vi "Settings Dialog.vi"(8 "error in (no error)":errorcluster, 11 "Settings In":T1={"Camera Configuration"={"Camera Index"=0}, "Logging Configuration"={"Log File Base Path"=path ""}, "XYZ Configuration"={"VISA resource name"="", "Timeout (3sec)"=0}, "DM Configuration"={"Selected Profile"="", "dm out"={"type"=0, "ID"=0, "size"=0, "@dummy control@"=0, "@dummy control@"=0, "@dummy control@"=0, "@dummy control@"=0, "lutName"=0}}, "Automation Configuration"={" Index"=0}, "V7001 Configuration"={" Index"=0}, "AOD Configuration"={"Physical Channel"="Dev1/ao0:1", "Maximum Value"=0.0, "Minimum Value"=1.0, "Update Rate"=192000.0}} {"AOD Configuration"."Update Rate" format="%0.2f"; "AOD Configuration"."Minimum Value" format="%0.2f"; "AOD Configuration"."Maximum Value" format="%0.2f"}) -> (0 "error out":errorcluster, 1 "Cancelled?":bool, 2 "UI Refresh Needed?":bool, 3 "Settings Out":T1={"Camera Configuration"={"Camera Index"=0}, "Logging Configuration"={"Log File Base Path"=path ""}, "XYZ Configuration"={"VISA resource name"="", "Timeout (3sec)"=0}, "DM Configuration"={"Selected Profile"="", "dm out"={"type"=0, "ID"=0, "size"=0, "@dummy control@"=0, "@dummy control@"=0, "@dummy control@"=0, "@dummy control@"=0, "lutName"=0}}, "Automation Configuration"={" Index"=0}, "V7001 Configuration"={" Index"=0}, "AOD Configuration"={"Physical Channel"="Dev1/ao0:1", "Maximum Value"=0.0, "Minimum Value"=1.0, "Update Rate"=192000.0}} {"AOD Configuration"."Update Rate" format="%0.2f"; "AOD Configuration"."Minimum Value" format="%0.2f"; "AOD Configuration"."Maximum Value" format="%0.2f"})   [LabVIEW 2015, in "Settings.lvlib"]
uses:
  Settings.lvlib
  <vilib>/Utility/xml.llb/Write to XML File(string).vi
  Camera/Camera Configuration.ctl
  Camera/Camera.lvlib
  Logging/Logging Configuration.ctl
  Logging/Logging.lvlib
  Settings.ctl
  XYZStage/XYZStage Configuration.ctl
  XYZStage/XYZStage.lvlib
  DM/DM Configuration.ctl
  DM/DM.lvlib
  Automation/Automation Configuration.ctl
  Automation/Automation.lvlib
  V7001/V7001 Configuration.ctl
  V7001/V7001.lvlib
  AOD/AOD Configuration.ctl
  AOD/AOD.lvlib
panel:
  in  "Cancel Button":bool
  in  "OK Button":bool
  in  "Log File Path":path
  in  "Signal Type":u16(ring) items=["Sine Wave", "Square with Noise"]
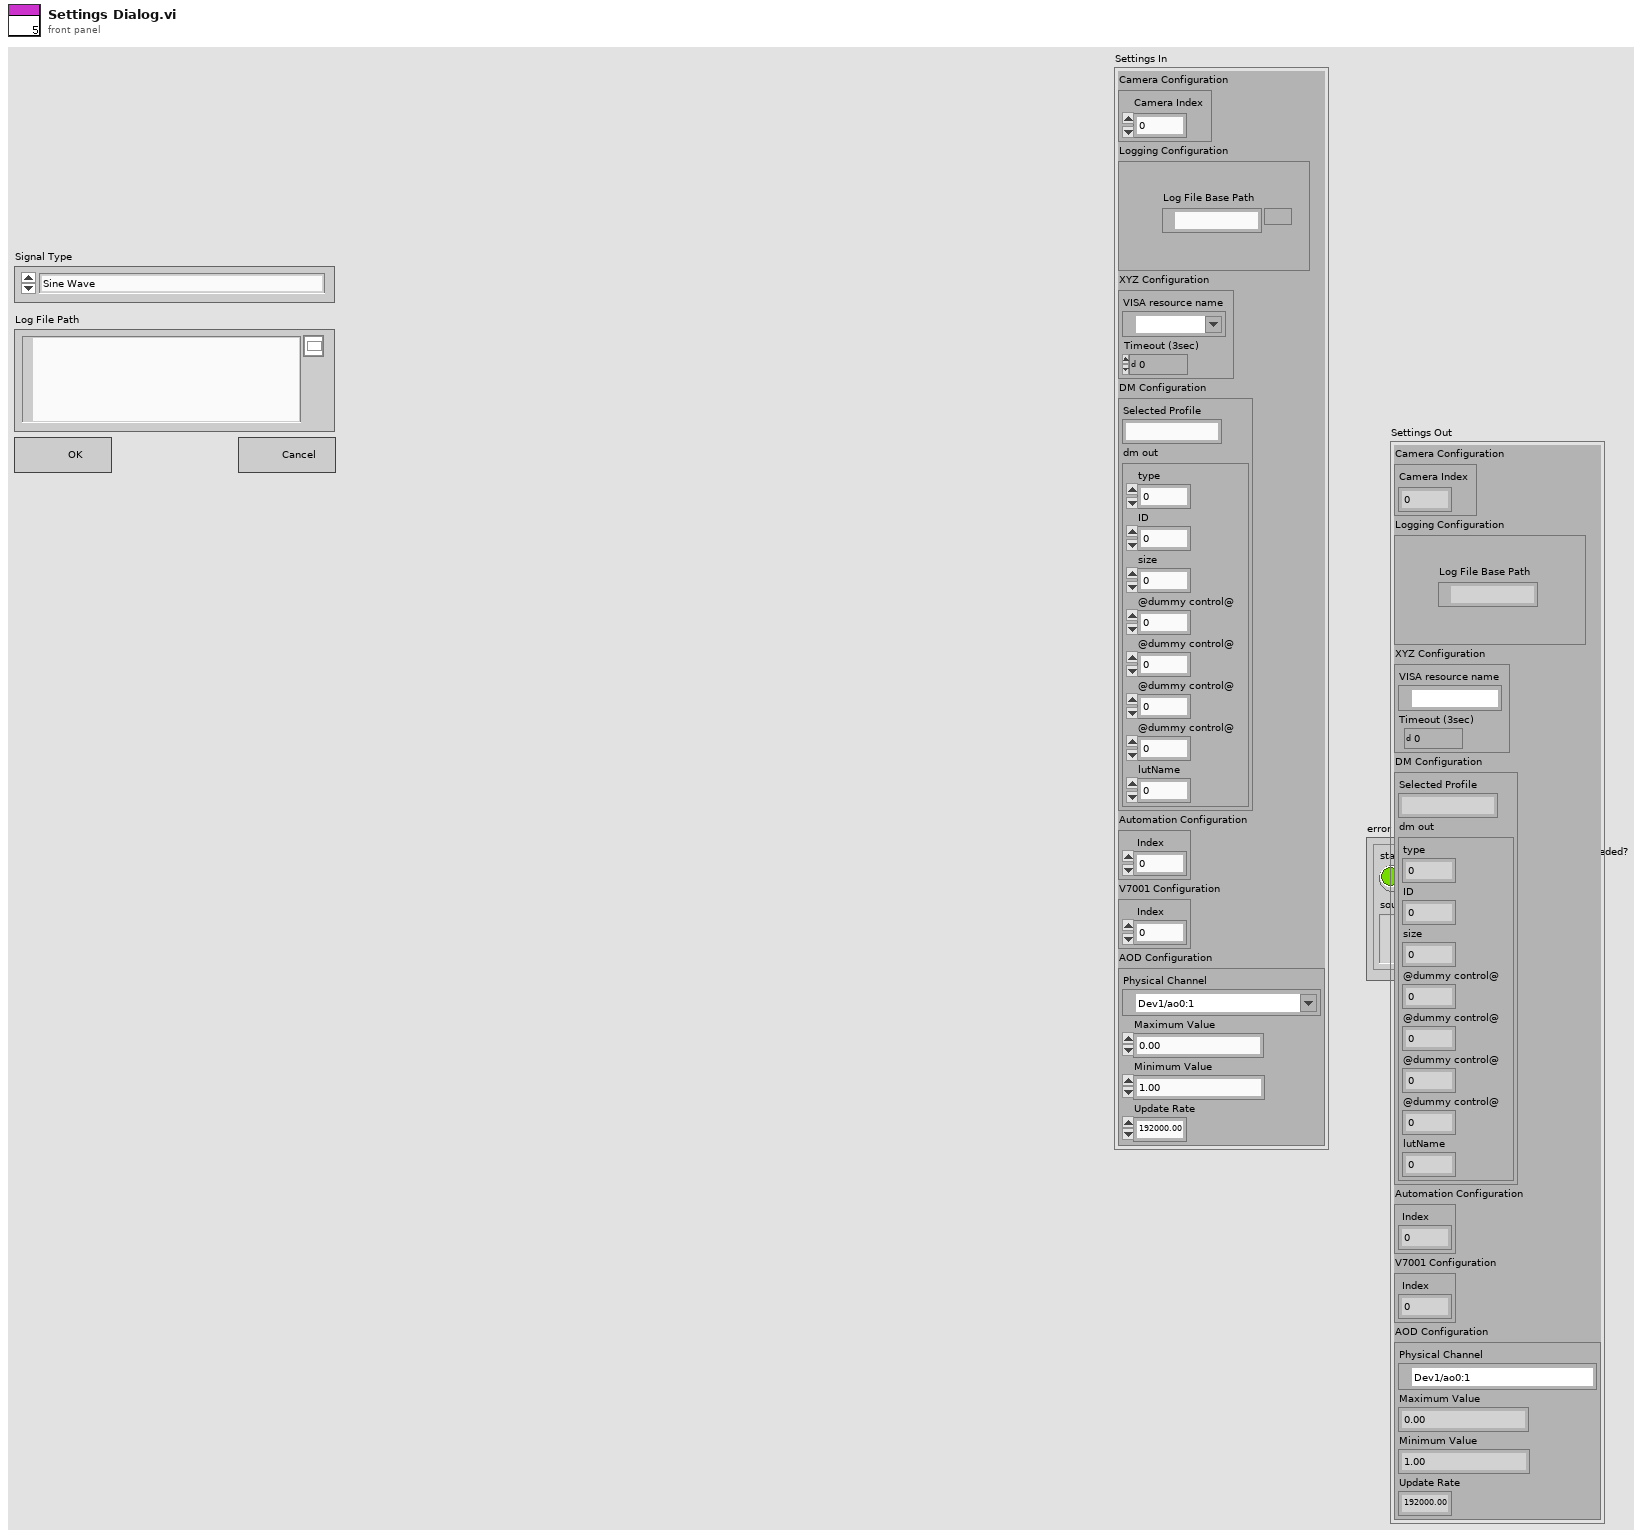
[diagram p1: front panel]
types:
  T1 = typedef "Settings.lvlib/Settings.ctl" = cluster{"Camera Configuration":T2, "Logging Configuration":T3, "XYZ Configuration":T4, "DM Configuration":T5, "Automation Configuration":T6, "V7001 Configuration":T7, "AOD Configuration":T8}
  T2 = typedef "Camera.lvlib/Camera Configuration.ctl" = cluster{"Camera Index":u32}
  T3 = typedef "Logging.lvlib/Logging Configuration.ctl" = cluster{"Log File Base Path":path}
  T4 = typedef "XYZStage.lvlib/XYZStage Configuration.ctl" = cluster{"VISA resource name":refnum<visa-resource-name>, "Timeout (3sec)":u32}
  T5 = typedef "DM.lvlib/DM Configuration.ctl" = cluster{"Selected Profile":string, "dm out":cluster{"type":i32, "ID":i32, "size":i32, "@dummy control@":i8, "@dummy control@":i8, "@dummy control@":i8, "@dummy control@":i8, "lutName":u64}}
  T6 = typedef "Automation.lvlib/Automation Configuration.ctl" = cluster{" Index":u32}
  T7 = typedef "V7001.lvlib/V7001 Configuration.ctl" = cluster{" Index":u32}
  T8 = typedef "AOD.lvlib/AOD Configuration.ctl" = cluster{"Physical Channel":tag, "Maximum Value":dbl, "Minimum Value":dbl, "Update Rate":dbl}
  T9 = typedef "Acquisition.lvlib/Signal Type.ctl" = enum16{"Sine Wave", "Square with Noise"}
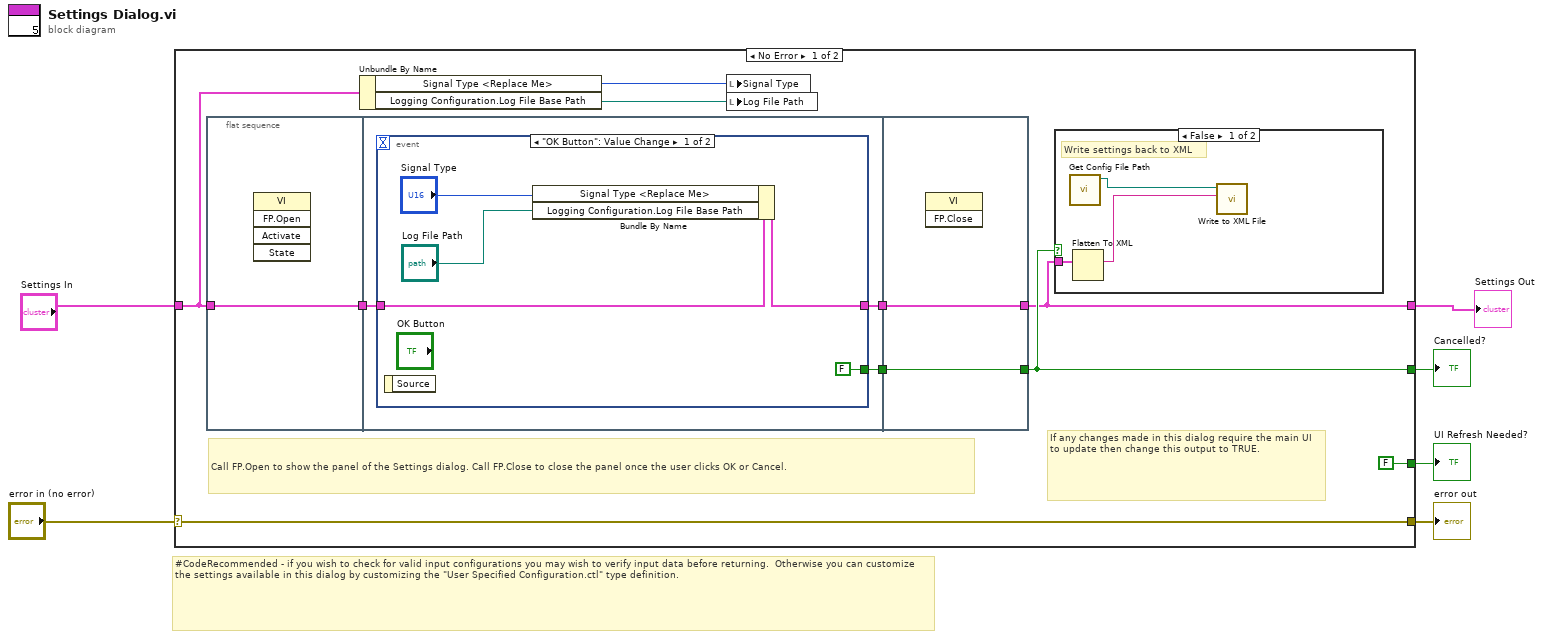
[diagram p0: block diagram]
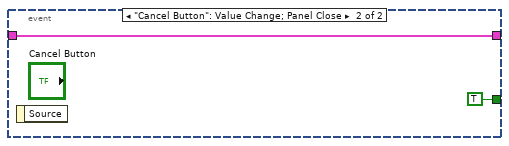
[diagram p2: hidden frame]
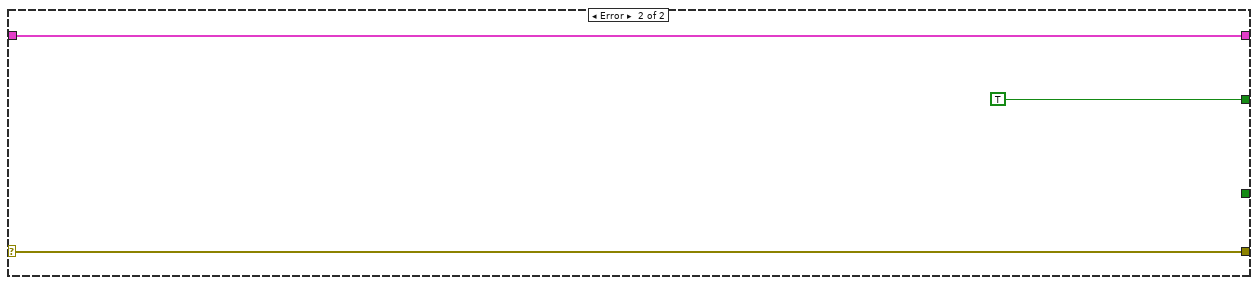
[diagram p4: hidden frame]
diagram:
  # "#CodeRecommended - if you wish to check for valid input configurations you may wish to verify input data before returning.  Otherwise you can customize the settings available in this dialog by customizing the \"User Specified Configuration.ctl\" type definition."
  n1 = case shown="No Error" "error in (no error)" {
    selector: "error in (no error)" -> [w16 w35]
    tunnel: [w16 w35] -> w5
    tunnel: "Settings In" -> [w12 w34]
    tunnel: [w13 w34] -> w1
    tunnel: [FALSE ("UI Refresh Needed?") _] -> w4
    tunnel: [w14 TRUE ("UI Refresh Needed?")] -> w3
    frame No Error {
      # "Call FP.Open to show the panel of the Settings dialog. Call FP.Close to close the panel once the user clicks OK or Cancel."
      # "If any changes made in this dialog require the main UI to update then change this output to TRUE."
      n2 = flat-sequence {
        tunnel: w12 -> [w17]
        tunnel: [w17] -> w9
        tunnel: w9 -> [w18]
        tunnel: [w20] -> w8
        tunnel: [w19] -> w7
        tunnel: [w28] -> w13
        tunnel: [w29] -> w14
        tunnel: w8 -> [w29]
        tunnel: w7 -> [w28]
        frame #0 {
          n3 = invoke class="VI" method="FP.Open"() -> ()  [unwired: 5 in, 5 out]
        }
        frame #1 {
          n4 = event shown="[0] \"OK Button\": Value Change" {
            selector: _ -> [_ _]
            dyn-events: _ -> [_ _]
            timeout: _ -> [_ _]
            tunnel: [w23 w27] -> w19
            tunnel: w18 -> [w24 w27]
            tunnel: [FALSE ("UI Refresh Needed?") TRUE ("UI Refresh Needed?")] -> w20
            event "OK Button": Value Change {
              n5 = event-data() -> ()  [unwired: 1 in, 1 out]
              n6 = Bundle By Name(cluster=w24, "Signal Type <Replace Me>"="Signal Type", "Logging Configuration.Log File Base Path"="Log File Path") -> (w23:T1)
            }
            event "Cancel Button": Value Change; Panel Close {
              n7 = event-data() -> ()  [unwired: 1 in, 1 out]
            }
          }
        }
        frame #2 {
          n8 = invoke class="VI" method="FP.Close"() -> ()  [unwired: 3 in, 3 out]
        }
      }
      n9 = Unbundle By Name(w12) -> ("Signal Type <Replace Me>"=w11:T9, "Logging Configuration.Log File Base Path"=w10:path)
      n10 = local write "Signal Type"(w11) -> ()
      n11 = local write "Log File Path"(w10) -> ()
      n12 = case shown="False" w14 {
        tunnel: w13 -> [w32 _]
        frame False {
          # "Write settings back to XML"
          n13 = call "Get Config File Path.vi"() -> ("XML File Path"=w30:path)  [unwired: 10 in, 1 out]
          n14 = Flatten To XML(anything=w32) -> (xml string=w31:string)
          n15 = call-poly <vilib>:"Write to XML File.vi"("XML Input"=w31, "XML File Path"=w30) -> ()  [unwired: 7 in, 3 out]
        }
        frame True {
        }
      }
    }
    frame Error {
    }
  }
  "UI Refresh Needed?" <- w4
  "error out" <- w5
  "Cancelled?" <- w3
  "Settings Out" <- w1
